vi "Stacked Secuence Local.vi"() -> ()   [LabVIEW 2020]
panel:
  in  "Boolean":bool
  in  "Send Data":string
  in  "Variador":dbl(knob) scale=0.0..100.0
  out "String 2":string
  out "Thermometer":dbl(slide) scale=0.0..100.0
  out "Boolean 2":bool
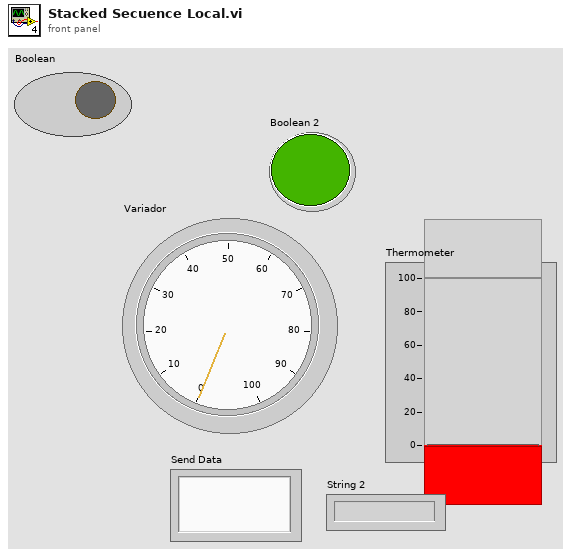
[diagram p1: front panel]
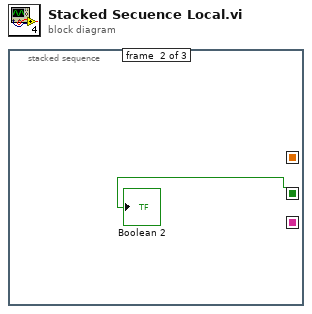
[diagram p0: block diagram]
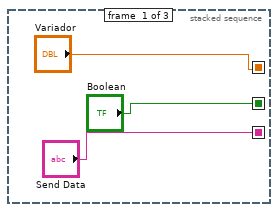
[diagram p2: hidden frame]
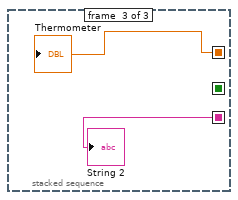
[diagram p3: hidden frame]
diagram:
  n1 = stacked-sequence {
    seq-local: ["Send Data" _ _] -> [_ _ w5]
    seq-local: ["Boolean" _ _] -> [_ w4 _]
    seq-local: ["Variador" _ _] -> [_ _ w6]
    frame #0 {
    }
    frame #1 {
      "Boolean 2" <- w4
    }
    frame #2 {
      "Thermometer" <- w6
      "String 2" <- w5
    }
  }
